vi "NotificationGetReportDatesRequest_Name.vi"() -> (1 "MessageName":string)   [LabVIEW 2017]
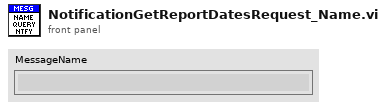
[diagram p1: front panel]
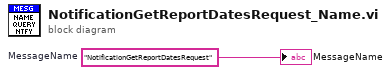
[diagram p0: block diagram]
diagram:
  w1 = "NotificationGetReportDatesRequest"  # MessageName
  "MessageName" <- w1
